vi "initialize Session Data.vi"(0 "Session in":refnum<class "niRFSTS Sequence Flow.lvclass">, 11 "error in":errorcluster) -> (4 "Session out":refnum<class "niRFSTS Sequence Flow.lvclass">, 15 "error out":errorcluster)   [LabVIEW 2018, in "niRFSTS Sequence Flow.lvclass"]
uses:
  niRFSTS Sequence Flow.lvclass
  Plugins/Sequence Automation Session.lvlibp/Sequence Automation Session.lvclass
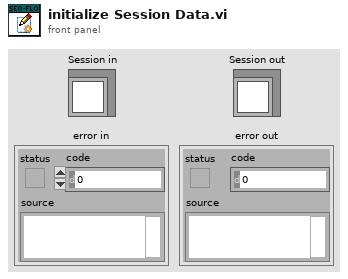
[diagram p1: front panel]
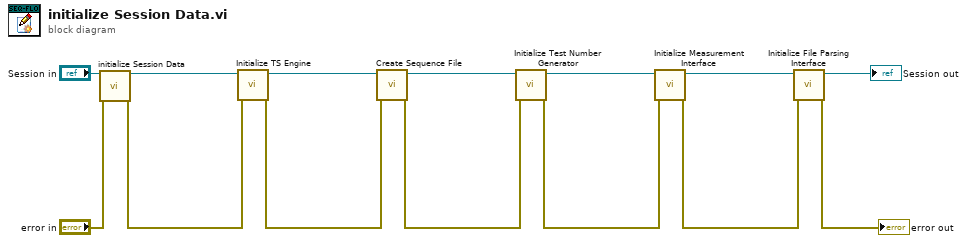
[diagram p0: block diagram]
diagram:
  n1 = call-parent "initialize Session Data.vi"("OBJ - Session in"="Session in", "error in"="error in") -> ("OBJ - Session out"=w12:refnum<class "niRFSTS Sequence Flow.lvclass">, "error out"=w11:errorcluster)  [unwired: 12 in]
  n2 = call-dynamic "Initialize TS Engine.vi"("error in (no error)"=w11, "niRFSTS Sequence Flow in"=w12) -> ("error out"=w9:errorcluster, "niRFSTS Sequence Flow out"=w10:refnum<class "niRFSTS Sequence Flow.lvclass">)  [unwired: 8 in]
  n3 = call-dynamic "Create Sequence File.vi"("error in (no error)"=w9, "niRFSTS Sequence Flow in"=w10) -> ("error out"=w4:errorcluster, "niRFSTS Sequence Flow out"=w8:refnum<class "niRFSTS Sequence Flow.lvclass">)  [unwired: 8 in]
  n4 = call-dynamic "Initialize Test Number Generator.vi"("error in (no error)"=w4, "niRFSTS Sequence Flow in"=w8) -> ("error out"=w3:errorcluster, "niRFSTS Sequence Flow out"=w7:refnum<class "niRFSTS Sequence Flow.lvclass">)  [unwired: 8 in]
  n5 = call-dynamic "Initialize Measurement Interface.vi"("error in (no error)"=w3, "niRFSTS Sequence Flow in"=w7) -> ("error out"=w2:errorcluster, "niRFSTS Sequence Flow out"=w6:refnum<class "niRFSTS Sequence Flow.lvclass">)  [unwired: 8 in]
  n6 = call-dynamic "Initialize File Parsing Interface.vi"("error in (no error)"=w2, "niRFSTS Sequence Flow in"=w6) -> ("error out"=→"error out":errorcluster, "niRFSTS Sequence Flow out"=→"Session out":refnum<class "niRFSTS Sequence Flow.lvclass">)  [unwired: 8 in]
